vi "HEAD_ACK_TYPE.vi"(9 "Record":i32, 11 "GBD":string) -> (3 "output cluster":T1 caption="HEAD" {"FirstPos" format="%<%x %.3X>T"; "Stop" format="%<%x %.3X>T"; "Trig" format="%<%x %.3X>T"; "Start" format="%<%x %.3X>T"})   [LabVIEW 2017]
uses:
  Amp_Param.ctl
panel:
  out "Data":string[](array[string])
  # "ALL"
  # "GBD"
  # "CSV"
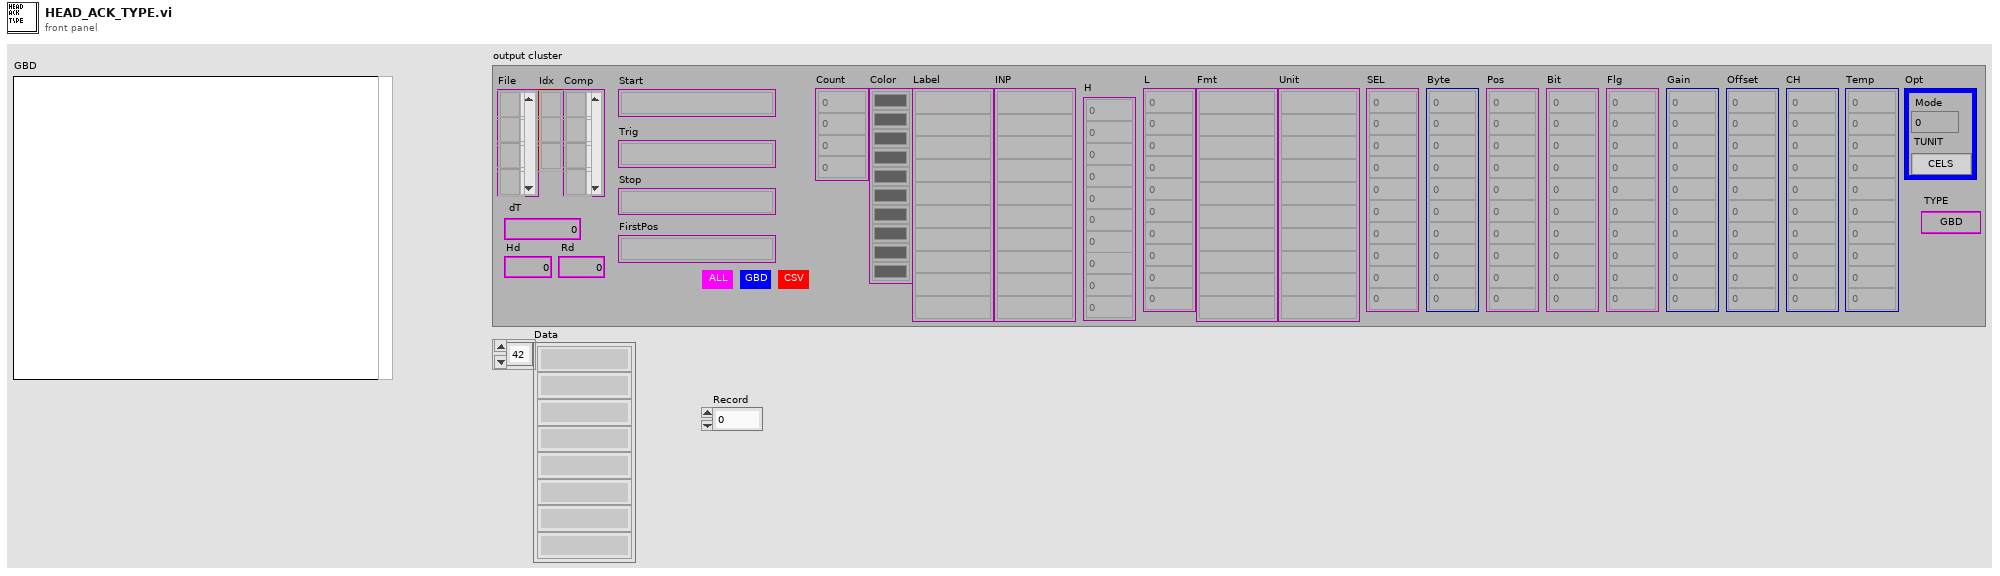
[diagram p1: front panel]
types:
  T1 = typedef "Amp_Param.ctl" = cluster{"File":refnum<file>[], "Idx":refnum<file>[], "dT":dbl, "Hd":i32, "Rd":i32, "Start":timestamp[], "Trig":timestamp[], "Stop":timestamp[], "FirstPos":timestamp[], "Count":i64[], "Color":u32[], "Label":string[], "INP":string[], "H":dbl[], "L":dbl[], "Fmt":string[], "Unit":string[], "SEL":i32[], "Byte":i32[], "Pos":i32[], "Bit":i32[], "Flg":i32[], "Gain":dbl[], "Offset":dbl[], "CH":i32[], "Opt":cluster{"Mode":i32, "TUNIT":enum16{"CELS", "FAHR"}}, "TYPE":enum16{"GBD", "CSV"}, "Comp":refnum<file>[], "Temp":i32[]}
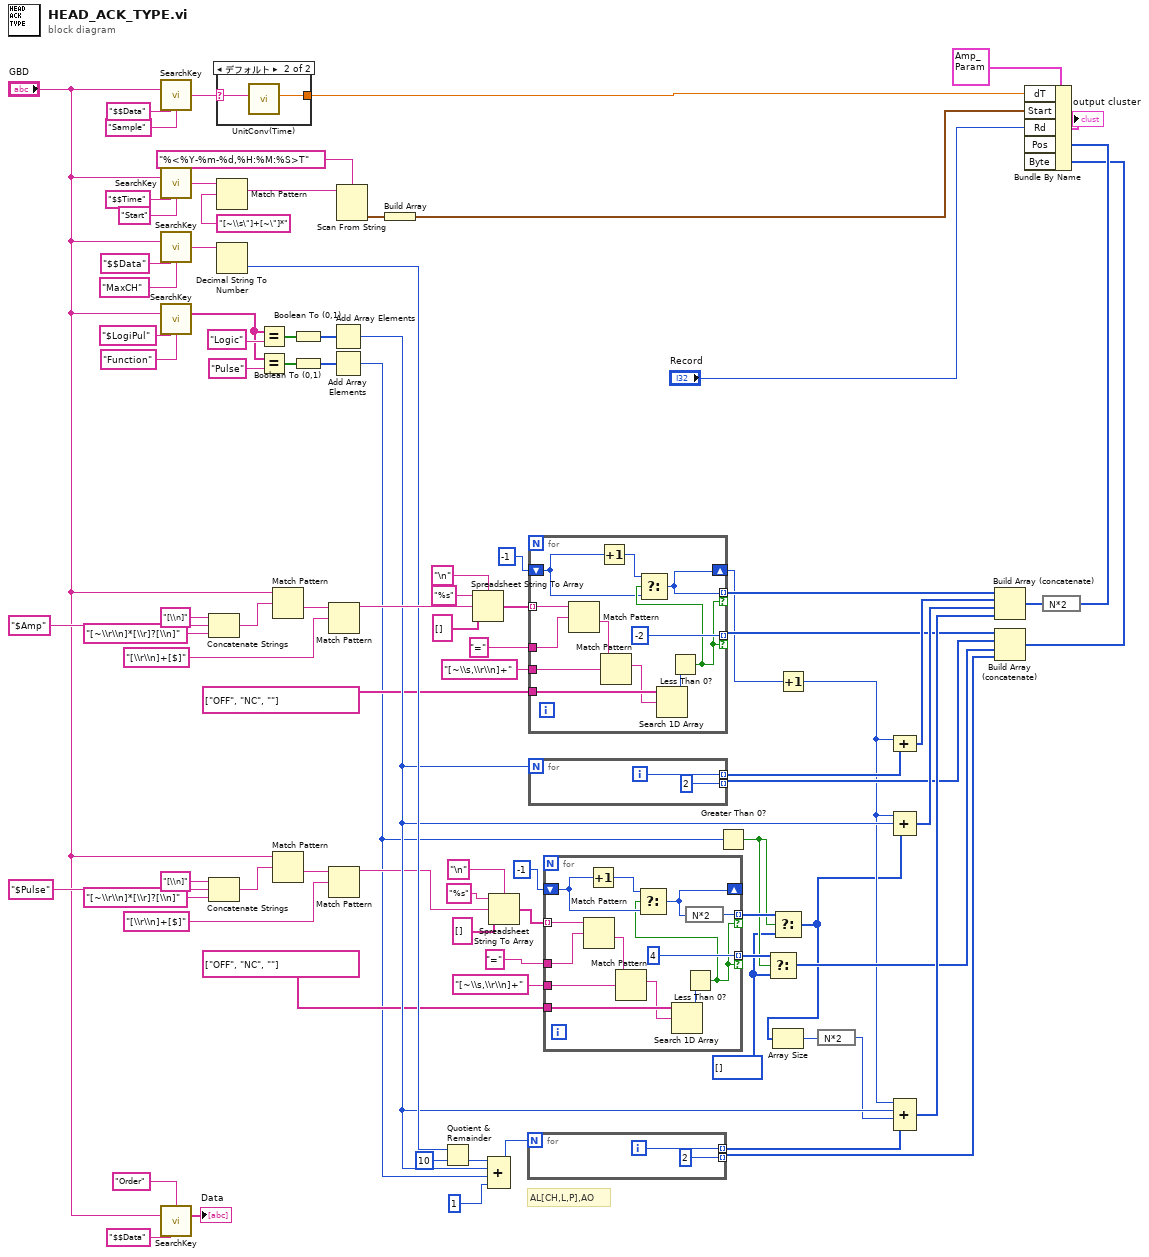
[diagram p0: block diagram]
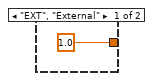
[diagram p2: hidden frame]
diagram:
  w10 = i32[] []
  # "AL[CH,L,P],AO"
  n1 = call "SearchKey.vi"("In"="GBD", "KEY1"="$$Data", "KEY2"="Sample") -> ("String"=w38:string)  [unwired: 12 out]
  n2 = call "SearchKey.vi"("In"="GBD", "KEY1"="$$Time", "KEY2"="Start") -> ("String"=w48:string)  [unwired: 12 out]
  n3 = call "SearchKey.vi"("In"="GBD", "KEY1"="$$Data", "KEY2"="MaxCH") -> ("String"=w72:string)  [unwired: 12 out]
  n4 = call "SearchKey.vi"("In"="GBD", "KEY1"="$LogiPul", "KEY2"="Function") -> ("Data"=w76:string[])  [unwired: 12 out]
  n5 = call "SearchKey.vi"("In"="GBD", "KEY1"="$$Data", "KEY2"="Order") -> ("Data"=→"Data":string[])  [unwired: 12 out]
  n6 = Concatenate Strings("[\\n]" ("string"), "$Amp" ("string"), "[~\\r\\n]*[\\r]?[\\n]" ("string")) -> (w83:string)
  n7 = Concatenate Strings("[\\n]" ("string"), "$Pulse" ("string"), "[~\\r\\n]*[\\r]?[\\n]" ("string")) -> (w59:string)
  n8 = case shown="デフォルト" w38 {
    selector: w38 -> [_ w92]
    tunnel: [1.0 ("NumOUT") w93] -> w37
    frame "EXT", "External" {
    }
    frame Default {
      n9 = call "UnitConv(Time).vi"("St IN"=w92) -> ("NumOUT"=w93:dbl)  [unwired: 3 in, 5 out]
    }
  }
  n10 = Match Pattern(string=w48, regular expression="[~\\s\"]+[~\"]*") -> (match substring=w43:string)  [unwired: 4 out]
  n11 = Decimal String To Number(string=w72) -> (number=w53:i32)  [unwired: 2 in, 1 out]
  n12 = Equal?(x=w76, y="Logic") -> (x = y?=w89:bool[])
  n13 = Equal?(x=w76, y="Pulse") -> (x = y?=w85:bool[])
  n14 = Match Pattern(string="GBD", regular expression=w83) -> (after substring=w79:string)  [unwired: 4 out]
  n15 = Match Pattern(string="GBD", regular expression=w59) -> (after substring=w63:string)  [unwired: 4 out]
  n16 = Boolean To (0,1)(Boolean=w89) -> (0, 1=w88:i16[])
  n17 = Boolean To (0,1)(Boolean=w85) -> (0, 1=w86:i16[])
  n18 = Match Pattern(string=w79, regular expression="[\\r\\n]+[$]" ("string")) -> (before substring=w65:string)  [unwired: 4 out]
  n19 = Match Pattern(string=w63, regular expression="[\\r\\n]+[$]" ("string")) -> (before substring=w19:string)  [unwired: 4 out]
  n20 = Add Array Elements(numeric array=w88) -> (sum=w51:i16)
  n21 = Add Array Elements(numeric array=w86) -> (sum=w15:i16)
  n22 = Scan From String(format string="%<%Y-%m-%d,%H:%M:%S>T", input string=w43) -> (output 1=w42:timestamp)  [unwired: 3 in, 3 out]
  n23 = Build Array(w42) -> (w41:timestamp[])
  n24 = Quotient & Remainder(x=w53, y=10) -> (floor(x/y)=w34:i32)  [unwired: 1 out]
  n25 = Spreadsheet String To Array(delimiter (Tab)="\n" ("format string"), format string="%s", spreadsheet string=w65, array type (2D Dbl)=string[] []) -> (array=w68:string[])
  n26 = Compound Arithmetic op=ADD(w34, w51, w15, 1) -> (w50:i32)
  n27 = Spreadsheet String To Array(delimiter (Tab)="\n" ("format string"), format string="%s", spreadsheet string=w19, array type (2D Dbl)=string[] []) -> (array=w21:string[])
  n28 = for {
    N: w50 -> [_]
    tunnel: [w95] -> w54 mode=indexing
    tunnel: [2] -> w31 mode=indexing
    i -> [w95]
  }
  n29 = for {
    tunnel: w68 -> [w107] mode=indexing
    tunnel: "=" ("regular expression") -> [w105]
    tunnel: "[~\\s,\\r\\n]+" ("regular expression") -> [w104]
    tunnel: [w96] -> w6 mode=indexing if=w99
    tunnel: [-2] -> w33 mode=indexing if=w99
    tunnel: string[] ["OFF", "NC", ""] -> [w102]
    shift-right: [w96] -> w3
    shift-left: -1 -> [w97]
    n30 = Match Pattern(string=w107, regular expression=w105) -> (after substring=w106:string)  [unwired: 4 out]
    n31 = Increment(x=w97) -> (x+1=w98:i32)
    n32 = Match Pattern(string=w106, regular expression=w104) -> (match substring=w101:string)  [unwired: 4 out]
    n33 = Search 1D Array(1D array=w102, element=w101) -> (index of element=w100:i32)  [unwired: 1 in]
    n34 = Less Than 0?(x=w100) -> (x < 0?=w99:bool)
    n35 = Select(t=w98, s=w99, f=w97) -> (s? t:f=w96:i32)
  }
  n36 = for {
    N: w51 -> [_]
    tunnel: [w109] -> w58 mode=indexing
    tunnel: [2] -> w32 mode=indexing
    i -> [w109]
  }
  n37 = for {
    tunnel: w21 -> [w122] mode=indexing
    tunnel: "=" ("regular expression") -> [w120]
    tunnel: "[~\\s,\\r\\n]+" ("regular expression") -> [w119]
    tunnel: [w111] -> w12 mode=indexing if=w113
    tunnel: [4] -> w13 mode=indexing if=w113
    tunnel: string[] ["OFF", "NC", ""] -> [w117]
    shift-right: [w112] -> _
    shift-left: -1 -> [w114]
    n38 = Match Pattern(string=w122, regular expression=w120) -> (after substring=w121:string)  [unwired: 4 out]
    n39 = Increment(x=w114) -> (x+1=w110:i32)
    n40 = Match Pattern(string=w121, regular expression=w119) -> (match substring=w116:string)  [unwired: 4 out]
    n41 = Search 1D Array(1D array=w117, element=w116) -> (index of element=w115:i32)  [unwired: 1 in]
    n42 = Less Than 0?(x=w115) -> (x < 0?=w113:bool)
    n43 = Select(t=w110, s=w113, f=w114) -> (s? t:f=w112:i32)
    n44 = expression code="N*2"(w112) -> (w111:i32)
  }
  n45 = Greater Than 0?(x=w15) -> (x > 0?=w11:bool)
  n46 = Select(t=w13, s=w11, f=w10) -> (s? t:f=w14:i32[])
  n47 = Select(t=w12, s=w11, f=w10) -> (s? t:f=w1:i32[])
  n48 = Array Size(array=w1) -> (size(s)=w2:i32)
  n49 = Increment(x=w3) -> (x+1=w4:i32)
  n50 = expression code="N*2"(w2) -> (w5:i32)
  n51 = Compound Arithmetic op=ADD(w4, w58) -> (w57:i32[])
  n52 = Compound Arithmetic op=ADD(w4, w51, w1) -> (w56:i32[])
  n53 = Compound Arithmetic op=ADD(w4, w51, w5, w54) -> (w49:i32[])
  n54 = Build Array (concatenate)(w6, w57, w56, w49) -> (w55:i32[])
  n55 = Build Array (concatenate)(w33, w32, w14, w31) -> (w30:i32[])
  n56 = expression code="N*2"(w55) -> (w35:i32[])
  n57 = Bundle By Name(cluster=T1 {"File"=[], "Idx"=[], "dT"=0.0, "Hd"=0, "Rd"=0, "Start"=[], "Trig"=[], "Stop"=[], "FirstPos"=[], "Count"=[], "Color"=[], "Label"=[], "INP"=[], "H"=[], "L"=[], "Fmt"=[], "Unit"=[], "SEL"=[], "Byte"=[], "Pos"=[], "Bit"=[], "Flg"=[], "Gain"=[], "Offset"=[], "CH"=[], "Opt"={"Mode"=0, "TUNIT"=enum."CELS"}, "TYPE"=enum."GBD", "Comp"=[], "Temp"=[]} ("HEAD"), "dT"=w37, "Start"=w41, "Rd"="Record", "Pos"=w35, "Byte"=w30) -> (→"output cluster":T1)
